vi "SigSyn (G3)-Create.vi"(6 "Rep Num":i32, 8 "error in (no error)":errorcluster, 9 "Npts":i32, 10 "Sampling Rate (Hz)":dbl, 11 "Stimulus Channel":T1 {"Filter"."Stages"."IIR Filter"."Forward Coefficients" format="%.4f"; "Filter"."Stages"."IIR Filter"."Reverse Coefficients" format="%.4f"}) -> (0 "error out":errorcluster, 1 "Sampling Rate (out)":dbl, 2 "Waveform":dbl[](graph), 3 "Stimulus Channel out":T1 {"Filter"."Stages"."IIR Filter"."Forward Coefficients" format="%.4f"; "Filter"."Stages"."IIR Filter"."Reverse Coefficients" format="%.4f"})   [LabVIEW 2020]
uses:
  XControls/Stimulus Channel (G3)/Full Stimulus Channel Data.ctl
  XControls/Waveform XControls/Waveform (G3)/Waveform Data.ctl
  Waveform VIs/Waveform Enum (V3).ctl
  XControls/Waveform XControls/Tone (G3)/Tone.Properties.ctl
  Waveform VIs/Pulse Train VIs/Pulse Train Params.ctl
  Waveform VIs/Pulse Train VIs/Pulse Polarity.ctl
  Waveform VIs/Pulse Train VIs/PT-Continuous State.ctl
  Waveform VIs/Noise VIs/Noise (G3).ctl
  Waveform VIs/Noise VIs/Noise (G3).Properties.ctl
  Waveform VIs/Noise VIs/Noise (G3).Data.ctl
  Waveform VIs/File VIs/StimFile-Params.ctl
  Waveform VIs/FM Sweep VIs/FM Sweep Params.ctl
  Waveform VIs/Chirp Train VIs/Chirp Train.ctl
  Waveform VIs/Chirp Train VIs/Chirp Train Params.ctl
  Waveform VIs/Complex Tone VIs/CT-Params.ctl
  Waveform VIs/Complex Tone VIs/CT-Phase Enum.ctl
  Waveform VIs/Complex Tone VIs/CT-Runtime Data.ctl
  XControls/Waveform XControls/FM Tone/Data.ctl
  XControls/Waveform XControls/Vowel/Vowel.Properties.ctl
  Waveform VIs/Ramp VIs/Ramp.Properties.ctl
  XControls/Filter (G3)/Filter Data.ctl
  XControls/Filter (G3)/Filter Type.ctl
  Filter VIs/Filter-Bandwidth Units.ctl
  Controls/Burst XCtl/Burst Data.ctl
  XControls/Level (G3)/Level Data.ctl
  XControls/Level (G3)/Level Units (G3).ctl
  XControls/Advanced Options (G3)/Advanced Options (G3).ctl
  Modulation VIs/SAM VIs/SAM Params.ctl
  Typedefs/Destination.ctl
  Controls/Level XCtl/Level Units.ctl
  XControls/Filter (G3)/Filter (G3).xctl
  XControls/Level (G3)/Level (G3).xctl
  Controls/Burst XCtl/Burst Control.xctl
  XControls/Waveform XControls/Waveform (G3)/Waveform (G3).xctl
  XControls/Advanced Options (G3)/Advanced Options (G3).xctl
  XControls/Stimulus Channel (G3)/Stimulus Channel (G3).xctl
  XControls/Waveform XControls/Tone (G3)/Tone (G3).xctl
  XControls/Waveform XControls/FM Tone/FM Tone.xctl
  XControls/Waveform XControls/Vowel/Vowel.xctl
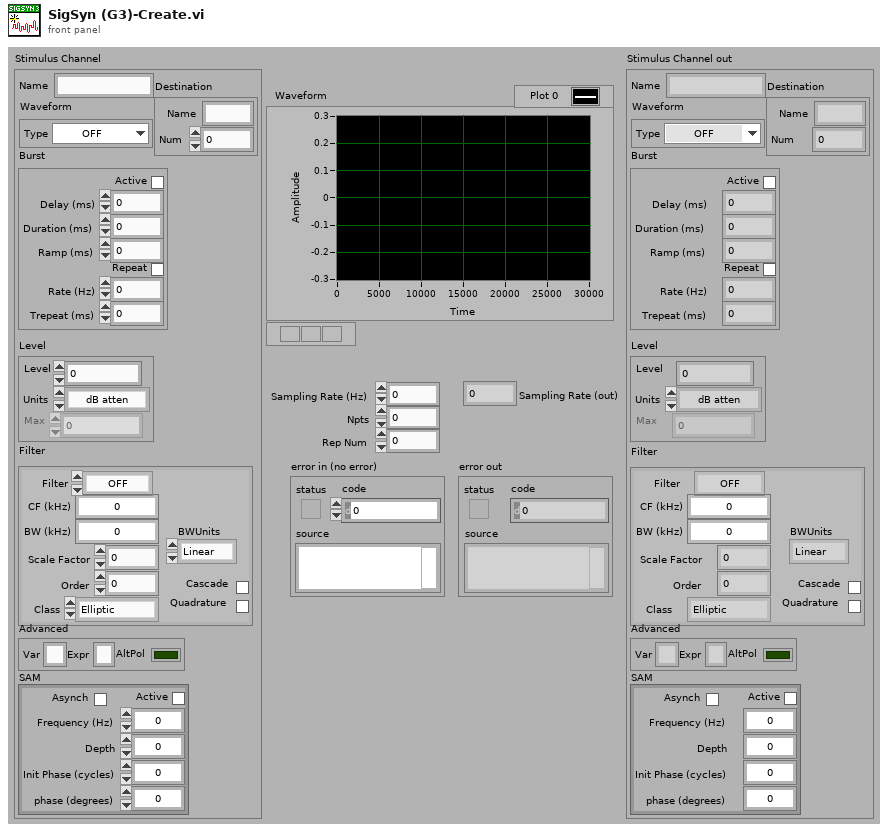
[diagram p1: front panel]
types:
  T1 = typedef "Stimulus Channel (G3).xctl/Full Stimulus Channel Data.ctl" = cluster{"Waveform":T2, "Filter":T21, "Burst":T24, "Level":T25, "Name":string, "Advanced":T27, "SAM":T28, "Destination":T29}
  T2 = typedef "Waveform (G3).xctl/Waveform Data.ctl" = cluster{"Type":T3, "Tone":T4, "Pulse Train":T5, "Noise":T8, "File":T11, "FMSweep":T12, "Chirp Train":T13, "Complex Tone":cluster{"Params":T15, "Data":T17}, "FM":T18, "Vowel":T19, "Ramp":T20}
  T3 = typedef "Waveform Enum (V3).ctl" = enum16{"OFF", "Tone", "Noise", "Pulse Train", "File", "FM Sweep", "Chirp Train", "Complex Tone", "FM Tone", "Vowel", "Ramp"}
  T4 = typedef "Tone (G3).xctl/Tone.Properties.ctl" = cluster{"Frequency (kHz)":dbl, "Phase (cycles)":dbl, "Random phase":bool}
  T5 = typedef "Pulse Train Params.ctl" = cluster{"Pulse width (us)":dbl, "Pulse rate (Hz)":dbl, "Gap (ms)":dbl, "Polarity":T6, "PT State":T7, "Asynch":bool}
  T6 = typedef "Pulse Polarity.ctl" = enum16{"POS", "NEG", "POS-NEG", "NEG-POS"}
  T7 = typedef "PT-Continuous State.ctl" = cluster{"Template":dbl[], "Nperiod":i32, "Index":i32, "Pulse Rate (Hz)":dbl, "Phase (cycles)":dbl, "Noff":i32}
  T8 = typedef "Noise (G3).ctl" = cluster{"Properties":T9, "Data":T10}
  T9 = typedef "Noise (G3).Properties.ctl" = cluster{"InvFilt":bool, "Aweight":bool, "Seed":i32, "Tokens":i32, "Brickwall":bool}
  T10 = typedef "Noise (G3).Data.ctl" = cluster{"TokenNum":i32}
  T11 = typedef "StimFile-Params.ctl" = cluster{"Filename":path, "Signal":dbl[], "Channel":i32, "stream":bool, "offset":i32, "nreps":i32, "loops":i32, "Randomize":bool, "order":i32[], "Seed":i32, "Tokens":i32}
  T12 = typedef "FM Sweep Params.ctl" = cluster{"Rate (oct/s)":dbl, "Fmin (Hz)":dbl, "Fmax (Hz)":dbl, "Ramp (ms)":dbl, "Linear":bool}
  T13 = typedef "Chirp Train.ctl" = cluster{"Params":T14, "Data":cluster{"WF":dbl[]}}
  T14 = typedef "Chirp Train Params.ctl" = cluster{"Fmin (kHz)":dbl, "Fmax (kHz)":dbl, "Compensate":bool, "Duration (ms)":dbl}
  T15 = typedef "CT-Params.ctl" = cluster{"F0 (Hz)":dbl, "Band":cluster{"Flow (Hz)":dbl, "Fhigh (Hz)":dbl}, "Phase":T16, "Min F0 (Hz)":dbl, "Max F0 (Hz)":dbl, "ContinRandPhase":bool, "Max peak factor":dbl, "Max mod depth":dbl, "MinHarmNum":i32, "MaxHarmNum":i32, "Level Mode":enum16{"per component", "overall rms"}, "% jitter":dbl}
  T16 = typedef "CT-Phase Enum.ctl" = enum16{"Cosine", "Random", "Alternating"}
  T17 = typedef "CT-Runtime Data.ctl" = cluster{"Ncomp":i32, "MinHarm":i32, "Phase":dbl[], "Amplitude":dbl[], "Npts/frame":i32, "Last F0":dbl, "Fmin":dbl, "Fmax":dbl, "Lslope":dbl, "randphase":bool, "overall rms":bool, "fmult":dbl[], "jittered":bool}
  T18 = typedef "FM Tone.xctl/Data.ctl" = cluster{"Carrier (kHz)":dbl, "ModRate (Hz)":dbl, "Depth (Hz)":dbl, "Phase (cycles)":dbl}
  T19 = typedef "Vowel.xctl/Vowel.Properties.ctl" = cluster{"Freqs":string, "Set level":enum16{"Total", "Per component"}, "Freq":dbl[], "weights":dbl[]}
  T20 = typedef "Ramp.Properties.ctl" = cluster{"Duration (ms)":dbl}
  T21 = typedef "Filter (G3).xctl/Filter Data.ctl" = cluster{"Type":T22, "CF (kHz)":dbl, "BW (kHz)":dbl, "Cascade":bool, "Quadrature":bool, "Scale Factor":dbl, "Stages":cluster{"IIR Filter":cluster{"filter structure":enum32{"IIR 2nd Order", "IIR 4th Order"}, "Reverse Coefficients":dbl[], "Forward Coefficients":dbl[]}, "State":dbl[]}[], "Class":enum16{"Elliptic", "Butterworth"}, "Order":i32, "BWUnits":T23}
  T22 = typedef "Filter (G3).xctl/Filter Type.ctl" = enum16{"OFF", "Lowpass", "Highpass", "Bandpass", "Bandstop"}
  T23 = typedef "Filter-Bandwidth Units.ctl" = enum16{"Linear", "Octaves", "Min-Max"}
  T24 = typedef "Burst Control.xctl/Burst Data.ctl" = cluster{"Active":bool, "Delay (ms)":dbl, "Duration (ms)":dbl, "Ramp (ms)":dbl, "Rate (Hz)":dbl, "Trepeat (ms)":dbl, "Repeat":bool}
  T25 = typedef "Level (G3).xctl/Level Data.ctl" = cluster{"Level":dbl, "Units":T26, "Max":dbl, "Data":cluster{"Multiplier":dbl, "Cal File":path, "Cal":cluster{"Freq (Hz)":dbl[], "Mag (dB SPL)":dbl[], "Phase (deg)":dbl[]}, "audiogram":path}}
  T26 = typedef "Level (G3).xctl/Level Units (G3).ctl" = enum16{"dB atten", "dB SPL", "dB re 1 Vrms", "dB V/Hz½", "mW", "dB HL", "Volts", "dB mW"}
  T27 = typedef "Advanced Options (G3).xctl/Advanced Options (G3).ctl" = cluster{"AltPol":bool, "Var":string, "Expr":string}
  T28 = typedef "SAM Params.ctl" = cluster{"Active":bool, "Frequency (Hz)":dbl, "Depth":dbl, "Init Phase (cycles)":dbl, "phase (degrees)":dbl, "Asynch":bool}
  T29 = typedef "Destination.ctl" = cluster{"Name":string, "Num":i32}
  T30 = typedef "Level Units.ctl" = enum16{"dB atten", "dB SPL", "dB re 1 Vrms", "dB V/Hz½", "mW", "dB HL", "Volts", "dB mW"}
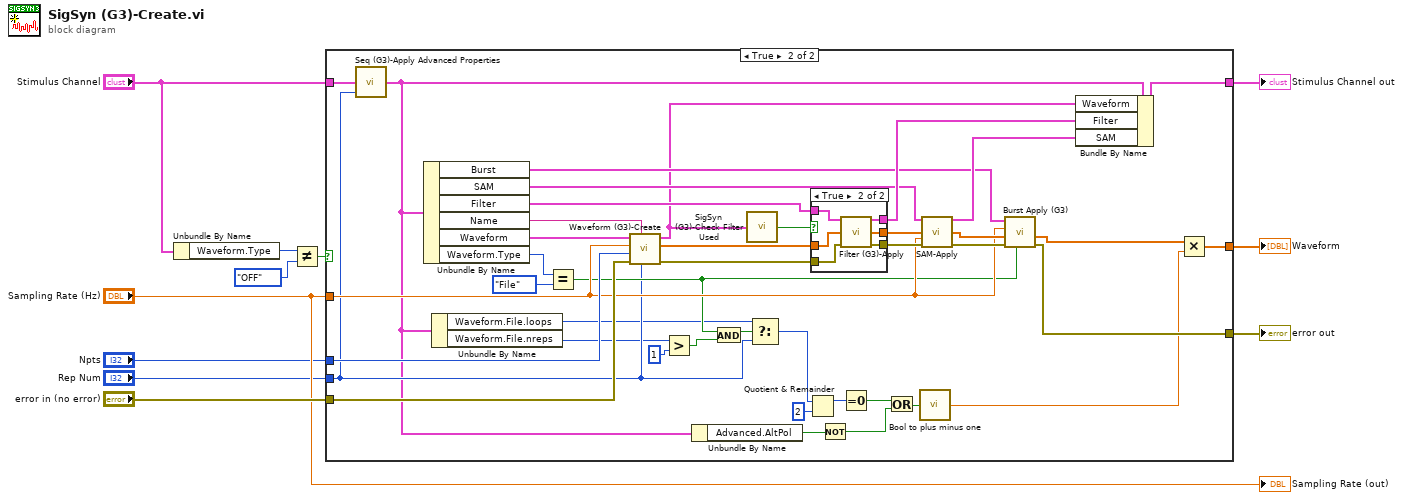
[diagram p0: block diagram]
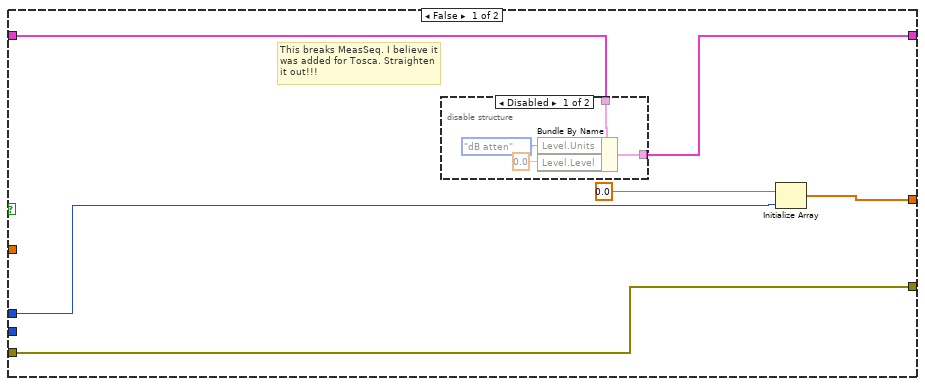
[diagram p2: hidden frame]
diagram:
  n1 = Unbundle By Name("Stimulus Channel") -> ("Waveform.Type"=w1:T3)
  n2 = Not Equal?(x=w1, y=Waveform_Enum_(V3)."OFF") -> (x != y?=w5:bool)
  n3 = case shown="True" w5 {
    tunnel: "error in (no error)" -> [w17 w63]
    tunnel: "Sampling Rate (Hz)" -> [_ w51]
    tunnel: [w17 w56] -> w10
    tunnel: "Npts" -> [w15 w62]
    tunnel: [w13 w44] -> w3
    tunnel: "Stimulus Channel" -> [w16 w39]
    tunnel: [w12 w57] -> w7
    tunnel: "Rep Num" -> [_ w31]
    frame False {
      # "This breaks MeasSeq. I believe it was added for Tosca. Straighten it out!!!"
      n4 = disable-structure shown="Disabled" {
        disable-tunnel: w16 -> [w21 w22]
        disable-tunnel: [w20 w22] -> w12
        frame Disabled {
          n5 = Bundle By Name(cluster=w21, "Level.Units"=Level_Units."dB atten" ("Level.Mode"), "Level.Level"=0.0) -> (w20:T1)
        }
        frame Enabled {
        }
      }
      n6 = Initialize Array(0.0 ("element"), w15) -> (w13:dbl[])
    }
    frame True {
      n7 = call "Seq (G3)-Apply Advanced Properties.vi"("Rep"=w31, "Stimulus Channel in"=w39) -> ("Stimulus Channel out"=w29:T1)  [unwired: 3 in]
      n8 = Unbundle By Name(w29) -> ("Burst"=w43:T24, "SAM"=w42:T28, "Filter"=w41:T21, "Name"=w38:string, "Waveform"=w37:T2, "Waveform.Type"=w36:T3)
      n9 = Unbundle By Name(w29) -> ("Waveform.File.loops"=w28:i32, "Waveform.File.nreps"=w26:i32)
      n10 = Equal?(x=w36, y=Waveform_Enum_(V3)."File") -> (x = y?=w32:bool)
      n11 = call "Waveform (G3)-Create.vi"("Rep Num"=w31, "Name"=w38, "error in (no error)"=w63, "Npts"=w62, "Sampling Rate (Hz)"=w51, "Waveform"=w37) -> ("error out"=w59:errorcluster, "Signal"=w60:dbl[], "Waveform out"=w33:T2)  [unwired: 3 in]
      n12 = Greater?(x=w26, y=1) -> (0:w24:bool)
      n13 = Unbundle By Name(w29) -> ("Advanced.AltPol"=w40:bool)
      n14 = And(x=w32, y=w24) -> (x .and. y?=w25:bool)
      n15 = call "SigSyn (G3)-Check Filter Used.vi"("Waveform in"=w33) -> ("Use filter"=w34:bool)
      n16 = Select(t=w28, s=w25, f=w31) -> (s? t:f=w30:i32)
      n17 = Quotient & Remainder(x=w30, y=2) -> (x-y*floor(x/y)=w48:i32)  [unwired: 1 out]
      n18 = case shown="True" w34 {
        tunnel: w60 -> [w65 w72]
        tunnel: w59 -> [w64 w71]
        tunnel: [w66 w70] -> w58
        tunnel: [w64 w69] -> w54
        tunnel: [w65 w68] -> w53
        tunnel: w41 -> [w66 w67]
        frame False {
        }
        frame True {
          n19 = call "Filter (G3)-Apply.vi"("Filter"=w67, "X"=w72, "error in (no error)"=w71) -> ("Filter out"=w70:T21, "Filtered X"=w68:dbl[], "error out"=w69:errorcluster)  [unwired: 10 in]
        }
      }
      n20 = Not(x=w40) -> (.not. x?=w46:bool)
      n21 = Equal To 0?(x=w48) -> (x = 0?=w47:bool)
      n22 = Or(x=w47, y=w46) -> (x .or. y?=w45:bool)
      n23 = call "Bool to plus minus one.vi"("Boolean"=w45) -> ("Numeric"=w27:dbl)
      n24 = call "SAM-Apply.vi"("SAM In"=w42, "X"=w53, "Sampling Rate (Hz)"=w51, "error in (no error)"=w54) -> ("SAM Out"=w50:T28, "Modulated X"=w52:dbl[], "error out"=w55:errorcluster)  [unwired: 9 in]
      n25 = call "Burst Apply (G3).vi"("Duplicate?"=w32, "error in (no error)"=w55, "Waveform in"=w52, "Sampling Rate (Hz)"=w51, "Burst"=w43) -> ("error out"=w56:errorcluster, "Gated waveform"=w61:dbl[])  [unwired: 5 in]
      n26 = Bundle By Name(cluster=w29, "Waveform"=w33, "Filter"=w58, "SAM"=w50) -> (w57:T1)
      n27 = Multiply(x=w61, y=w27) -> (x*y=w44:dbl[])
    }
  }
  "error out" <- w10
  "Waveform" <- w3
  "Stimulus Channel out" <- w7
  "Sampling Rate (out)" <- "Sampling Rate (Hz)"
